vi "Connect PV.vi"(8 "error in (no error)":errorcluster, 10 "PV URL":string, 11 "CS++DIMCommandMonitor in":refnum<class "CS++DIMCommandMonitor.lvclass">) -> (0 "error out":errorcluster, 3 "CS++DIMCommandMonitor out":refnum<class "CS++DIMCommandMonitor.lvclass">)   [LabVIEW 2016, in "CS++DIMMonitor.lvlib" / "CS++DIMCommandMonitor.lvclass"]
doc: "Open connection to process variable."
uses:
  CS++DIMCommandMonitor.lvclass
  C:/User/Brand/LVP/CSPP-Dev/Packages/CSPP_DIM/DIM_Monitor/CS++DIMMonitor.lvclass
  DIM_Monitor/CS++DIMMonitor.lvclass/CS++DIMMonitor.ctl
  DIM_Monitor/Write Services.vi
  DIM_Monitor/Write DIM IDs.vi
  DIM_Monitor/Read Services.vi
  DIM_Monitor/Read DIM IDs.vi
  DIM_Monitor/Read DIM Queue.vi
  DimLVEvent/LVDimInterface/LVDimInterface.dis_add_command_queue.vi
  DimLVEvent/LVDimInterface/LVDimInterface.lvlib
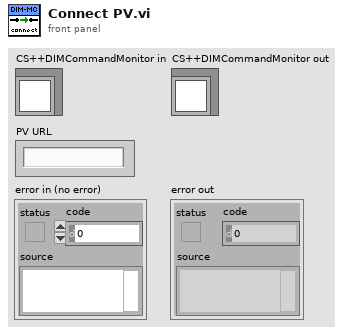
[diagram p1: front panel]
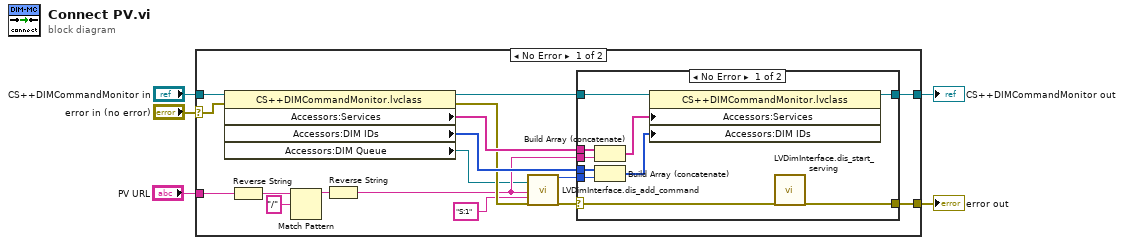
[diagram p0: block diagram]
diagram:
  n1 = case shown="No Error" "error in (no error)" {
    selector: "error in (no error)" -> [w14 w35]
    tunnel: "PV URL" -> [w19 _]
    tunnel: "CS++DIMCommandMonitor in" -> [w13 w36]
    tunnel: [w18 w36] -> w1
    tunnel: [w17 w35] -> w5
    frame No Error {
      n2 = property class="CS++DIMCommandMonitor.lvclass"(reference=w13, error in=w14) -> (reference out=w12:refnum<class "CS++DIMCommandMonitor.lvclass">, error out=w9:errorcluster, "Accessors:Services"=w16:string[], "Accessors:DIM IDs"=w15:i32[], "Accessors:DIM Queue"=w7:refnum<queue>)
      n3 = Reverse String(1:w19) -> (0:w21:string)
      n4 = Match Pattern(string=w21, regular expression="/" ("search string/char (-)")) -> (before substring=w20:string)  [unwired: 1 in, 3 out]
      n5 = Reverse String(1:w20) -> (0:w8:string)
      n6 = call-poly "LVDimInterface.dis_add_command.vi"("queueRef"=w7, "commandName"=w8, "typeDescriptor"="S:1", "error in (no error)"=w9) -> ("commandID"=w11:i32, "error out"=w10:errorcluster)  [unwired: 14 in]
      n7 = case shown="No Error" w10 {
        selector: w10 -> [w24 w33]
        tunnel: w12 -> [w28 w34]
        tunnel: [w27 w34] -> w18
        tunnel: w15 -> [w32 _]
        tunnel: w11 -> [w31 _]
        tunnel: w16 -> [w30 _]
        tunnel: w8 -> [w29 _]
        tunnel: [w23 w33] -> w17
        frame No Error {
          n8 = Build Array (concatenate)(w30, w29) -> (w26:string[])
          n9 = Build Array (concatenate)(w32, w31) -> (w25:i32[])
          n10 = property class="CS++DIMCommandMonitor.lvclass"(reference=w28, "Accessors:Services"=w26, "Accessors:DIM IDs"=w25) -> (reference out=w27:refnum<class "CS++DIMCommandMonitor.lvclass">)  [unwired: 1 in, 1 out]
          n11 = call "LVDimInterface.dis_start_serving.vi"("error in (no error)"=w24) -> ("error out"=w23:errorcluster)  [unwired: 17 in, 1 out]
        }
        frame Error {
        }
      }
    }
    frame Error {
    }
  }
  "error out" <- w5
  "CS++DIMCommandMonitor out" <- w1
